vi "Init Rx - Data.vi"(7 "Data Access in":refnum<class "Data Access Engine.lvclass">, 8 "error in (no error)":errorcluster, 11 "Parameters":variant) -> (0 "error out":errorcluster, 3 "Rx Loop Data":T1, 5 "Data Access out":refnum<class "Data Access Engine.lvclass">)   [LabVIEW 2019, in "UDP-Custom-Device Engine.lvlib"]
uses:
  UDP-Custom-Device Engine.lvlib
  Types/Engine - Rx Loop Data.ctl
  <vilib>/NI VeriStand/VeriStand Data/Byte Buffer/Byte Buffer.lvclass
  Types/Engine - General Resources.ctl
  <vilib>/NI VeriStand/VeriStand Data/Typedefs/Typedefs.Data Types.ctl
  Shared/Types/Shared - Duplex Settings.ctl
  Shared/Types/Shared - Header Details.ctl
  Shared/Types/Shared - Custom Header.ctl
  Types/Engine - Data Conversion Config.ctl
  <vilib>/NI VeriStand/VeriStand Data/Byte Buffer/Byte Buffer.Mapping.ctl
  Types/Engine - Rx Runtime Resources.ctl
  Types/Engine - Execution Config.ctl
  Shared/Types/Shared - Thread Management.ctl
  Types/Engine - Rx New Data Options Support.ctl
  Shared/Types/Shared - New Data Options.ctl
  Types/Engine - Rx Channel Refs.ctl
  <vilib>/NI/NIVS Inline Async API/_Data Access Engine/Data Access Engine/Types/Write.DVR.ctl
  <vilib>/NI/NIVS Inline Async API/_Data Access Engine/Access Type Classes/Write/Write.lvclass
  Types/Engine - Debug Resources.ctl
  <vilib>/NI/NIVS Inline Async API/_Data Access Engine/Data Access Engine/Data Access Engine.lvclass
  Shared/Types/Shared - Rx.PacketInfo.ctl
  Shared/Types/Shared - Channel Data Type.ctl
  Shared/Types/Shared - Buffered.PacketInfo.ctl
  Shared/Types/Shared - Pointer Encoding.ctl
  Shared/Types/Shared - Receive Buffer Options.ctl
  Shared/Types/Shared - Transmit Buffer Options.ctl
  <vilib>/NI/NIVS Inline Async API/_Data Access Engine/Data Access Engine/Methods/Write.Lookup.vi
  Shared/UDP-Custom-Device Shared.lvlib
  <vilib>/NI VeriStand/VeriStand Data/VeriStand Data.lvlib
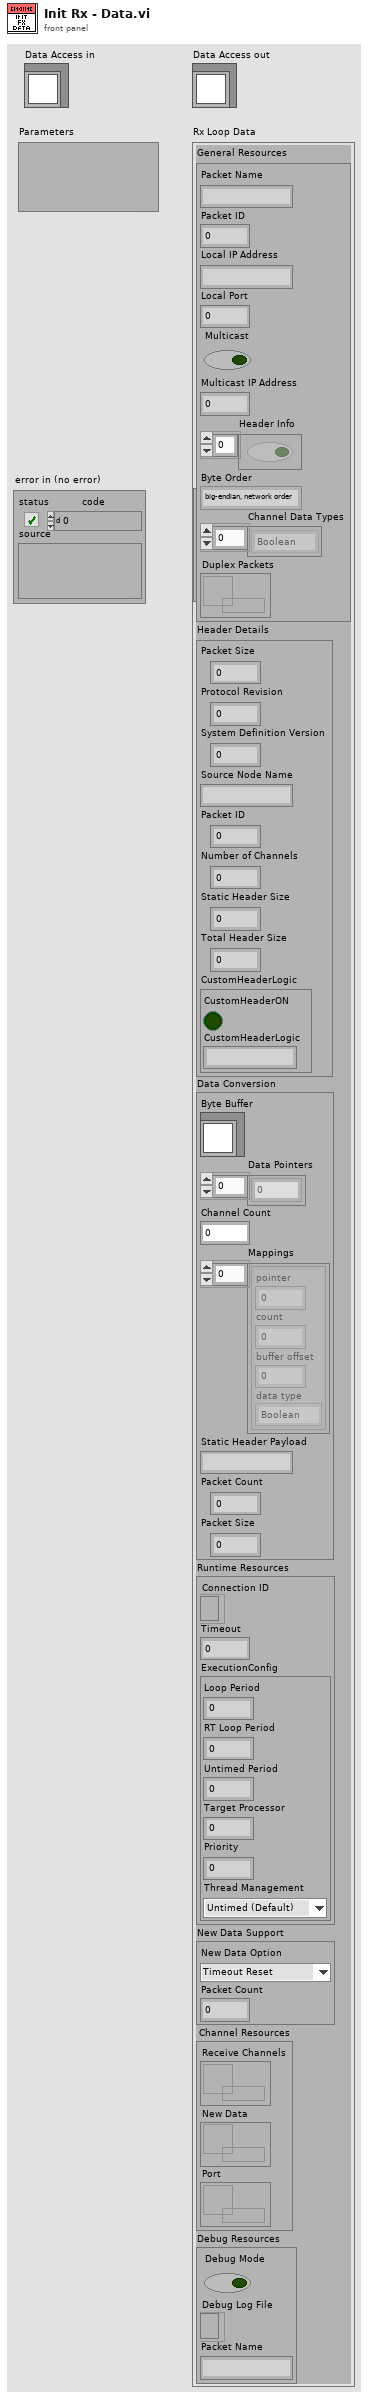
[diagram p1: front panel]
types:
  T1 = typedef "UDP-Custom-Device Engine.lvlib/Engine - Rx Loop Data.ctl" = cluster{"General Resources":T2, "Header Details":T4, "Data Conversion":T6, "Runtime Resources":T8, "New Data Support":T11, "Channel Resources":T13, "Debug Resources":T15}
  T2 = typedef "UDP-Custom-Device Engine.lvlib/Engine - General Resources.ctl" = cluster{"Packet Name":string, "Packet ID":i32, "Local IP Address":string, "Local Port":i32, "Multicast":bool, "Multicast IP Address":u32, "Header Info":bool[], "Byte Order":enum16{"big-endian, network order", "native, host order", "little-endian"}, "Channel Data Types":T3[], "Duplex Packets":refnum<data-value>}
  T3 = typedef "VeriStand Data.lvlib/Typedefs.Data Types.ctl" = enum16{"Boolean", "Single", "Double", "I8", "I16", "I32", "I64", "U8", "U16", "U32", "U64"}
  T4 = typedef "UDP-Custom-Device Shared.lvlib/Shared - Header Details.ctl" = cluster{"Packet Size":u16, "Protocol Revision":u8, "System Definition Version":u64, "Source Node Name":string, "Packet ID":u32, "Number of Channels":u32, "Static Header Size":u16, "Total Header Size":u16, "CustomHeaderLogic":T5}
  T5 = typedef "UDP-Custom-Device Shared.lvlib/Shared - Custom Header.ctl" = cluster{"CustomHeaderON":bool, "CustomHeaderLogic":string}
  T6 = typedef "UDP-Custom-Device Engine.lvlib/Engine - Data Conversion Config.ctl" = cluster{"Byte Buffer":refnum<class "Byte Buffer.lvclass">, "Data Pointers":u64[], "Channel Count":i32, "Mappings":T7[], "Static Header Payload":string, "Packet Count":dbl, "Packet Size":i32}
  T7 = typedef "VeriStand Data.lvlib/Byte Buffer.lvclass/Byte Buffer.Mapping.ctl" = cluster{"pointer":u64, "count":i64, "buffer offset":u64, "data type":T3}
  T8 = typedef "UDP-Custom-Device Engine.lvlib/Engine - Rx Runtime Resources.ctl" = cluster{"Connection ID":refnum<k16>, "Timeout":i32, "ExecutionConfig":T9}
  T9 = typedef "UDP-Custom-Device Engine.lvlib/Engine - Execution Config.ctl" = cluster{"Loop Period":i64, "RT Loop Period":i64, "Untimed Period":u32, "Target Processor":i32, "Priority":i32, "Thread Management":T10}
  T10 = typedef "UDP-Custom-Device Shared.lvlib/Shared - Thread Management.ctl" = enum16{"Untimed (Default)", "Timed (High Priority)"}
  T11 = typedef "UDP-Custom-Device Engine.lvlib/Engine - Rx New Data Options Support.ctl" = cluster{"New Data Option":T12, "Packet Count":dbl}
  T12 = typedef "UDP-Custom-Device Shared.lvlib/Shared - New Data Options.ctl" = enum16{"Timeout Reset", "Counter"}
  T13 = typedef "UDP-Custom-Device Engine.lvlib/Engine - Rx Channel Refs.ctl" = cluster{"Receive Channels":T14, "New Data":T14, "Port":T14}
  T14 = typedef "Data Access Engine.lvlib/Data Access Engine.lvclass/Write.DVR.ctl" = refnum<data-value>
  T15 = typedef "UDP-Custom-Device Engine.lvlib/Engine - Debug Resources.ctl" = cluster{"Debug Mode":bool, "Debug Log File":refnum<file>, "Packet Name":string}
  T16 = typedef "UDP-Custom-Device Shared.lvlib/Shared - Rx.PacketInfo.ctl" = cluster{"Packet Name":string, "Packet ID":i32, "Timeout":i32, "Rx IP Address":string, "Rx Port":u16, "Endianness":u16, "Multicast":bool, "Multicast IP Address":string, "Diagnostics En?":bool, "Debug Mode":bool, "Header Info":bool[], "Channel Data Types":T17[], "Buffered Packet Info":T18, "Duplex Packets":refnum<data-value>, "New Data Option":T12, "targetPriority":i16, "targetProcessor":i8, "Thread Management":T10}
  T17 = typedef "UDP-Custom-Device Shared.lvlib/Shared - Channel Data Type.ctl" = enum16{"Boolean", "Single", "Double", "I8", "I16", "I32", "I64", "U8", "U16", "U32", "U64"}
  T18 = typedef "UDP-Custom-Device Shared.lvlib/Shared - Buffered.PacketInfo.ctl" = cluster{"Buffer Size":i32, "External Buffer":bool, "Prepend Header":bool, "Is Buffered":bool, "Pointer Encoding":T19, "Rx Buffer Option":T20, "Tx Buffer Option":T21}
  T19 = typedef "UDP-Custom-Device Shared.lvlib/Shared - Pointer Encoding.ctl" = enum16{"Direct Encoding", "Conversion Encoding"}
  T20 = typedef "UDP-Custom-Device Shared.lvlib/Shared - Receive Buffer Options.ctl" = enum16{"Static Buffer", "Circular Buffer", "Circular Buffer + Size", "Internal Cache", "Internal Cache + Size", "Ping Pong", "Ping Pong + Size"}
  T21 = typedef "UDP-Custom-Device Shared.lvlib/Shared - Transmit Buffer Options.ctl" = enum16{"Static Buffer", "FIFO Buffer", "FIFO Buffer + Port"}
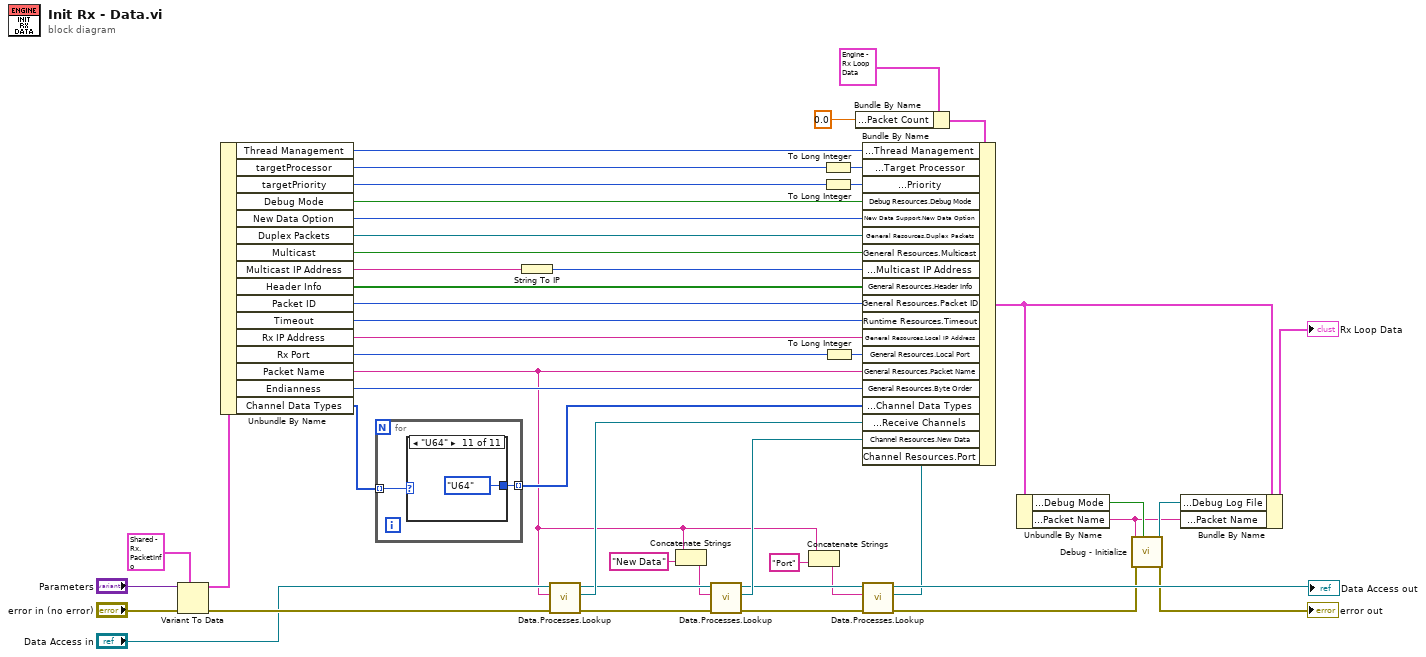
[diagram p0: block diagram]
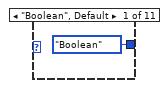
[diagram p2: hidden frame]
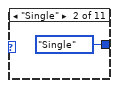
[diagram p3: hidden frame]
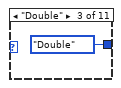
[diagram p4: hidden frame]
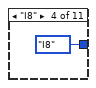
[diagram p5: hidden frame]
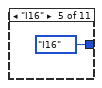
[diagram p6: hidden frame]
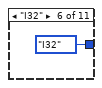
[diagram p7: hidden frame]
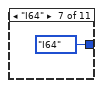
[diagram p8: hidden frame]
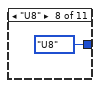
[diagram p9: hidden frame]
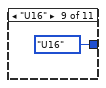
[diagram p10: hidden frame]
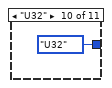
[diagram p11: hidden frame]
diagram:
  n1 = Variant To Data(error in="error in (no error)", type=T16 {"Packet Name"="", "Packet ID"=0, "Timeout"=0, "Rx IP Address"="", "Rx Port"=0, "Endianness"=0, "Multicast"=FALSE, "Multicast IP Address"="", "Diagnostics En?"=FALSE, "Debug Mode"=FALSE, "Header Info"=[], "Channel Data Types"=[], "Buffered Packet Info"={"Buffer Size"=0, "External Buffer"=FALSE, "Prepend Header"=FALSE, "Is Buffered"=FALSE, "Pointer Encoding"=enum."Direct Encoding", "Rx Buffer Option"=enum."Static Buffer", "Tx Buffer Option"=enum."Static Buffer"}, "Duplex Packets"=refnum, "New Data Option"=enum."Timeout Reset", "targetPriority"=1, "targetProcessor"=0, "Thread Management"=enum."Untimed (Default)"} ("Packet Info"), Variant="Parameters") -> (data=w46:T16, error out=w41:errorcluster)
  n2 = Unbundle By Name(w46) -> ("Thread Management"=w2:T10, "targetProcessor"=w6:i8, "targetPriority"=w5:i16, "Debug Mode"=w17:bool, "New Data Option"=w18:T12, "Duplex Packets"=w26:refnum<data-value>, "Multicast"=w29:bool, "Multicast IP Address"=w28:string, "Header Info"=w37:bool[], "Packet ID"=w42:i32, "Timeout"=w43:i32, "Rx IP Address"=w44:string, "Rx Port"=w45:u16, "Packet Name"=w20:string, "Endianness"=w38:u16, "Channel Data Types"=w36:T17[])
  n3 = for {
    tunnel: w36 -> [w51] mode=indexing
    tunnel: [w50] -> w35 mode=indexing
    n4 = case shown="\"U64\"" w51 {
      tunnel: [Typedefs.Data_Types."Boolean" ("data type") Typedefs.Data_Types."Single" ("data type") Typedefs.Data_Types."Double" ("data type") Typedefs.Data_Types."I8" ("data type") Typedefs.Data_Types."I16" ("data type") Typedefs.Data_Types."I32" ("data type") Typedefs.Data_Types."I64" ("data type") Typedefs.Data_Types."U8" ("data type") Typedefs.Data_Types."U16" ("data type") Typedefs.Data_Types."U32" ("data type") Typedefs.Data_Types."U64" ("data type")] -> w50
      frame "Boolean", Default {
      }
      frame "Single" {
      }
      frame "Double" {
      }
      frame "I8" {
      }
      frame "I16" {
      }
      frame "I32" {
      }
      frame "I64" {
      }
      frame "U8" {
      }
      frame "U16" {
      }
      frame "U32" {
      }
      frame "U64" {
      }
    }
  }
  n5 = String To IP(1:w28) -> (0:w27:u32)
  n6 = call-poly <vilib>:"Data.Processes.Lookup.vi"("error in (no error)"=w41, "Name"=w20, "Data Access API in"="Data Access in") -> ("error out"=w33:errorcluster, "Ref"=w39:T14, "Data Access API out"=w34:refnum<class "Data Access Engine.lvclass">)  [unwired: 5 in, 1 out]
  n7 = Concatenate Strings(w20, "New Data" ("Item GUID")) -> (w30:string)
  n8 = call-poly <vilib>:"Data.Processes.Lookup.vi"("error in (no error)"=w33, "Name"=w30, "Data Access API in"=w34) -> ("error out"=w23:errorcluster, "Ref"=w32:T14, "Data Access API out"=w25:refnum<class "Data Access Engine.lvclass">)  [unwired: 5 in, 1 out]
  n9 = Concatenate Strings(w20, "Port" ("Item GUID")) -> (w19:string)
  n10 = To Long Integer(number=w6) -> (32bit integer=w4:i32)
  n11 = To Long Integer(number=w5) -> (32bit integer=w3:i32)
  n12 = To Long Integer(number=w45) -> (32bit integer=w1:i32)
  n13 = Bundle By Name(cluster=T1 {"General Resources"={"Packet Name"="", "Packet ID"=0, "Local IP Address"="", "Local Port"=0, "Multicast"=FALSE, "Multicast IP Address"=0, "Header Info"=[], "Byte Order"=enum."big-endian, network order", "Channel Data Types"=[], "Duplex Packets"=refnum}, "Header Details"={"Packet Size"=0, "Protocol Revision"=0, "System Definition Version"=0, "Source Node Name"="", "Packet ID"=0, "Number of Channels"=0, "Static Header Size"=0, "Total Header Size"=0, "CustomHeaderLogic"={"CustomHeaderON"=FALSE, "CustomHeaderLogic"=""}}, "Data Conversion"={"Byte Buffer"=refnum, "Data Pointers"=[], "Channel Count"=0, "Mappings"=[], "Static Header Payload"="", "Packet Count"=0.0, "Packet Size"=0}, "Runtime Resources"={"Connection ID"=refnum, "Timeout"=0, "ExecutionConfig"={"Loop Period"=0, "RT Loop Period"=0, "Untimed Period"=0, "Target Processor"=0, "Priority"=0, "Thread Management"=enum."Untimed (Default)"}}, "New Data Support"={"New Data Option"=enum."Timeout Reset", "Packet Count"=0.0}, "Channel Resources"={"Receive Channels"=refnum, "New Data"=refnum, "Port"=refnum}, "Debug Resources"={"Debug Mode"=FALSE, "Debug Log File"=refnum, "Packet Name"=""}} ("Rx Loop Data"), "New Data Support.Packet Count"=0.0 ("Packet Count")) -> (w7:T1)
  n14 = call-poly <vilib>:"Data.Processes.Lookup.vi"("error in (no error)"=w23, "Name"=w19, "Data Access API in"=w25) -> ("error out"=w12:errorcluster, "Ref"=w22:T14, "Data Access API out"=→"Data Access out":refnum<class "Data Access Engine.lvclass">)  [unwired: 5 in, 1 out]
  n15 = Bundle By Name(cluster=w7, "Runtime Resources.ExecutionConfig.Thread Management"=w2, "Runtime Resources.ExecutionConfig.Target Processor"=w4, "Runtime Resources.ExecutionConfig.Priority"=w3, "Debug Resources.Debug Mode"=w17, "New Data Support.New Data Option"=w18, "General Resources.Duplex Packets"=w26, "General Resources.Multicast"=w29, "General Resources.Multicast IP Address"=w27, "General Resources.Header Info"=w37, "General Resources.Packet ID"=w42, "Runtime Resources.Timeout"=w43, "General Resources.Local IP Address"=w44, "General Resources.Local Port"=w1, "General Resources.Packet Name"=w20, "General Resources.Byte Order"=w38, "General Resources.Channel Data Types"=w35, "Channel Resources.Receive Channels"=w39, "Channel Resources.New Data"=w32, "Channel Resources.Port"=w22) -> (w14:T1)
  n16 = Unbundle By Name(w14) -> ("Debug Resources.Debug Mode"=w16:bool, "General Resources.Packet Name"=w10:string)
  n17 = call "Debug - Initialize.vi"("Debug Mode"=w16, "error in (no error)"=w12, "Packet Name"=w10) -> ("error out"=→"error out":errorcluster, "Debug Log File"=w15:refnum<file>)  [unwired: 7 in]
  n18 = Bundle By Name(cluster=w14, "Debug Resources.Debug Log File"=w15, "Debug Resources.Packet Name"=w10) -> (→"Rx Loop Data":T1)
